vi "DSF.Memory.Buffer.Config.Set Channel Types.vi"(8 "error in (no error)":errorcluster, 10 "channel types ptr":refnum<class "DSF.Engine.Memory.Pointer.DataType.lvclass">, 11 "Buffer Config in":refnum<class "DSF.Memory.Buffer.Config.lvclass">) -> (0 "error out":errorcluster, 3 "Buffer Config out":refnum<class "DSF.Memory.Buffer.Config.lvclass">)   [LabVIEW 2016, in "DSF.Engine.lvlib" / "DSF.Memory.Buffer.Config.lvclass"]
uses:
  DSF.Memory.Buffer.Config.lvclass
  Memory.Pointer/DSF.Engine.Memory.Pointer.DataType.lvclass
  DSF.Memory.Buffer.Config.lvclass/DSF.Memory.Buffer.Config.ctl
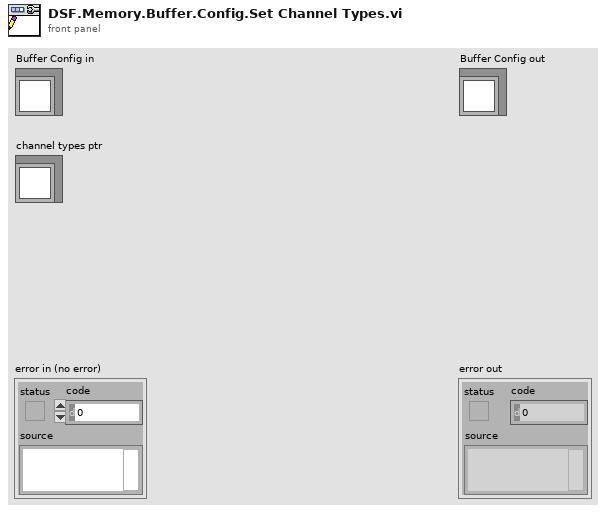
[diagram p1: front panel]
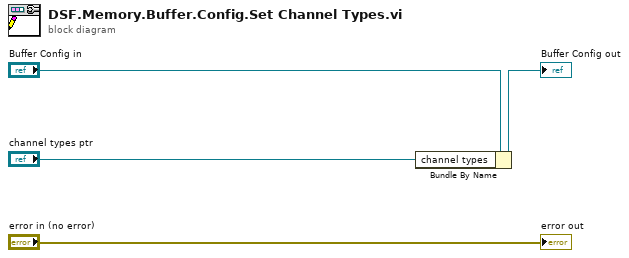
[diagram p0: block diagram]
diagram:
  n1 = Bundle By Name(cluster="Buffer Config in", "channel types"="channel types ptr") -> (→"Buffer Config out":refnum<class "DSF.Memory.Buffer.Config.lvclass">)
  "error out" <- "error in (no error)"
